vi "Zeile in Tabelle faerben.vi"(8 "error in (no error)":errorcluster caption="Fehler (Eingang, kein Fehler)", 9 "Fehler":bool[](array[boolean]), 11 "Ergebnisse":refnum<vi>) -> (0 "error out":errorcluster caption="Fehler (Ausgang)")   [LabVIEW 2020, in "Schedule Modul.lvlib"]
uses:
  Schedule Modul.lvlib
  Ergebnis Tabelle.ctl
  <vilib>/Utility/miscctls.llb/LVRowAndColumnTypeDef.ctl
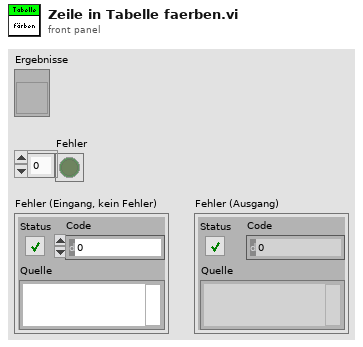
[diagram p1: front panel]
types:
  T1 = typedef "LVRowAndColumnTypeDef.ctl" = cluster{"Row":i32, "Column":i32}
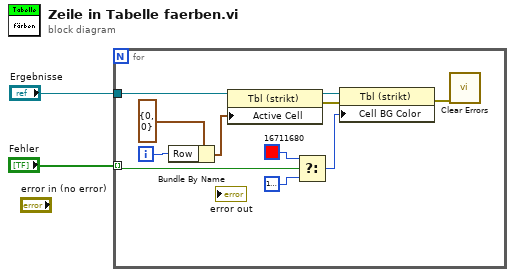
[diagram p0: block diagram]
diagram:
  n1 = for {
    tunnel: "Fehler" -> [w7] mode=indexing
    tunnel: "Ergebnisse" -> [w13]
    i -> [w11]
    n2 = Bundle By Name(cluster=T1 {"Row"=0, "Column"=0} ("Aktive Zelle:Aktive Zelle"), "Row"=w11) -> (w10:T1)
    n3 = property class="Tbl (strikt)"(reference=w13, "Active Cell"=w10) -> (reference out=w9:refnum<vi>, error out=w8:errorcluster)  [unwired: 1 in]
    n4 = Select(t=u32 16711680, s=w7, f=u32 16777216) -> (s? t:f=w4:u32)
    n5 = property class="Tbl (strikt)"(reference=w9, error in=w8, "Cell BG Color"=w4) -> (error out=w3:errorcluster)  [unwired: 1 out]
    n6 = call <vilib>:"Clear Errors.vi"("error in (no error)"=w3) -> ()  [unwired: 5 in, 2 out]
  }
